vi "Split Name and Message.vi"(10 "Delimiter (::::)":string="::::", 11 "Process Name/Message":string) -> (2 "Message":string, 3 "Process Name":string)   [LabVIEW 2020]
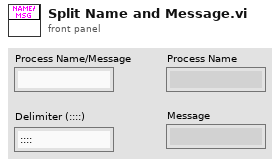
[diagram p1: front panel]
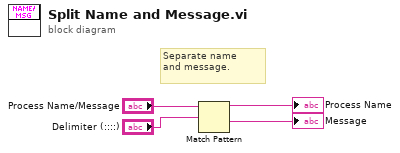
[diagram p0: block diagram]
diagram:
  # "Separate name\nand message."
  n1 = Match Pattern(string="Process Name/Message", regular expression="Delimiter (::::)") -> (before substring=→"Process Name":string, after substring=→"Message":string)  [unwired: 1 in, 2 out]
